vi "polarizer model.vi"(3 "output control":T1, 4 "data":variant, 5 "X":dbl[](array[numeric]), 6 "a":dbl[](array[numeric])) -> (0 "error out":errorcluster, 1 "f'(X,a)":dbl[][](array[numeric]), 2 "f(X,a)":dbl[](array[numeric]))   [LabVIEW 2023, in "Power Meter.lvlib"]
doc: "Sum of three Gaussians, plus DC offset."
uses:
  Power Meter/Power Meter.lvlib
  <vilib>/gmath/NumericalOptimization/LM_output select.ctl
  <vilib>/gmath/NI_Gmath.lvlib
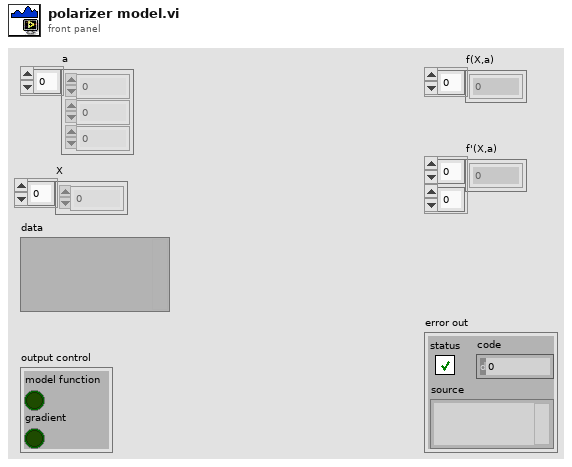
[diagram p1: front panel]
types:
  T1 = typedef "NI_Gmath.lvlib/LM_output select.ctl" = cluster{"model function":bool, "gradient":bool}
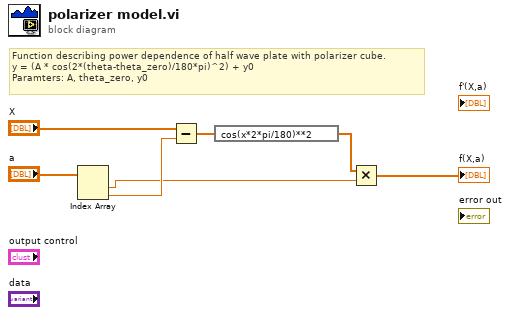
[diagram p0: block diagram]
diagram:
  # "Function describing power dependence of half wave plate with polarizer cube.\ny = (A * cos(2*(theta-theta_zero)/180*pi)^2) + y0\nParamters: A, theta_zero, y0"
  n1 = Index Array(array="a") -> (element #1=w4:dbl, element #2=w5:dbl)  [unwired: 2 in]
  n2 = Subtract(x="X", y=w5) -> (x-y=w2:dbl[])
  n3 = expression code="cos(x*2*pi/180)**2"(w2) -> (w1:dbl[])
  n4 = Multiply(x=w1, y=w4) -> (x*y=→"f(X,a)":dbl[])
